vi "Check bytes at port.vi"(8 "error in (no error)":errorcluster, 11 "ArduinoAISim in":refnum<class "ArduinoAISim.lvclass">) -> (0 "error out":errorcluster, 1 "Bytes available":bool, 2 "Number of Bytes at Serial Port":u32, 3 "ArduinoAISim out":refnum<class "ArduinoAISim.lvclass">)   [LabVIEW 2020, in "ArduinoAISim.lvclass"]
uses:
  ArduinoAISim.lvclass
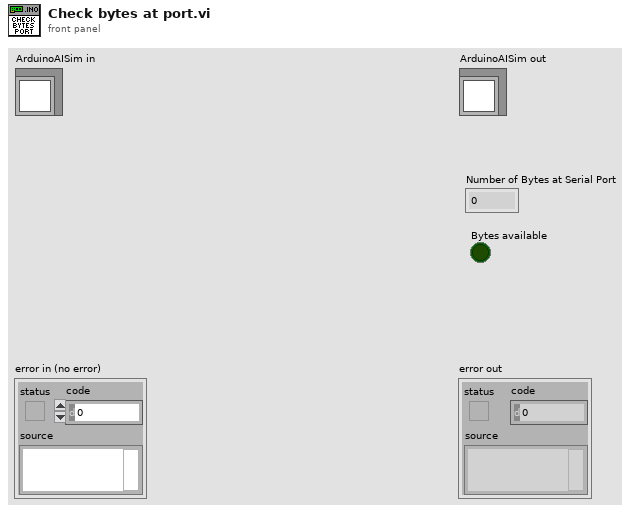
[diagram p1: front panel]
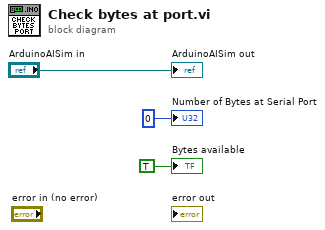
[diagram p0: block diagram]
diagram:
  "ArduinoAISim out" <- "ArduinoAISim in"
  "Number of Bytes at Serial Port" <- u32 0 ("Number of Bytes at Serial Port")
  "Bytes available" <- TRUE ("Bytes available")
